vi "HP 3458A Utility Output Format.vi"(5 "Output Format (0:ASCII)":T1(ring), 7 "Numbers of Reading (1)":i32=1, 9 "Input String":string) -> (4 "Output Data (ASCII)":dbl[](array[numeric]) format="%.4e", 6 "Output Data (Double Real)":dbl[](array[numeric]) format="%.4e", 8 "Output Data (Single Real)":sgl[](array[numeric]) format="%.4e", 10 "Output Data (Single Integer)":i16[](array[numeric]), 15 "Output Data (Double Integer)":i32[](array[numeric]) format="%.4e")   [LabVIEW 2014, in "SamplerPlugins.lvlib" / "HP3458aDMM.lvclass"]
doc: "This VI takes an input string and converts the string into numeric value according to the type of data that are being sent back. If the data type is not in ASCII characters, typecasting is then performed to changes the string into numeric type, with each number stored as an element in the output array."
uses:
  HP3458aDMM.lvclass
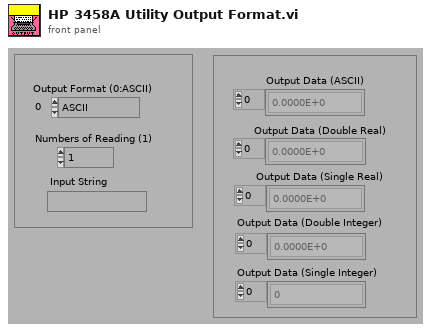
[diagram p1: front panel]
types:
  T1 = enum16{"ASCII", "Single Real", "Double Real", "Single Integer", "Double Integer"}
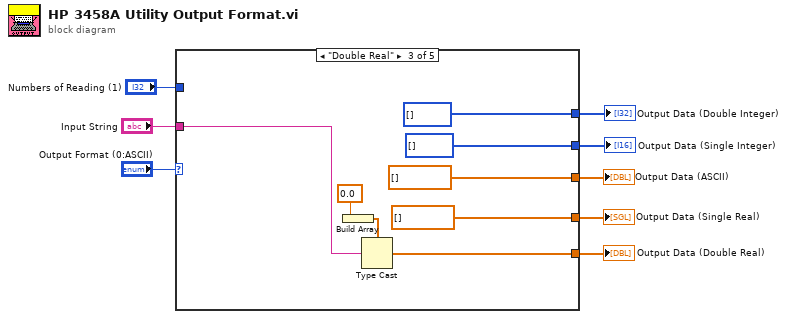
[diagram p0: block diagram]
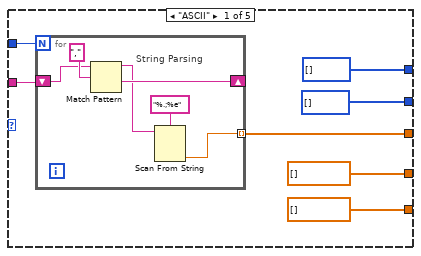
[diagram p2: hidden frame]
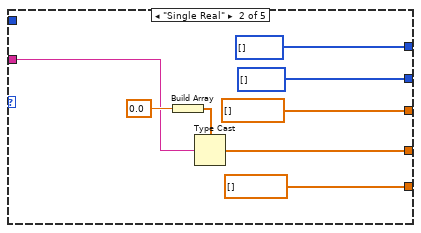
[diagram p3: hidden frame]
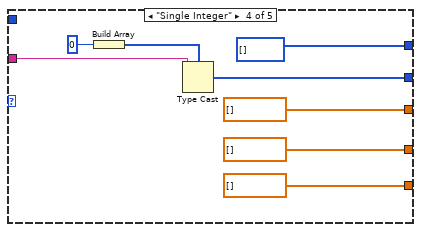
[diagram p4: hidden frame]
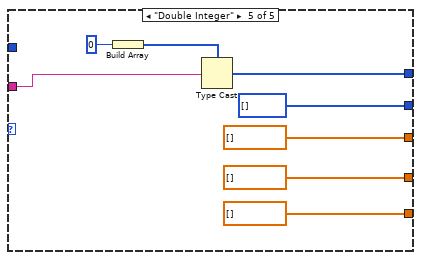
[diagram p5: hidden frame]
diagram:
  n1 = case shown="\"Double Real\"" "Output Format (0:ASCII)" {
    tunnel: [dbl[] [] dbl[] [] w35 dbl[] [] dbl[] []] -> w4
    tunnel: [sgl[] [] w26 sgl[] [] sgl[] [] sgl[] []] -> w5
    tunnel: [w15 dbl[] [] dbl[] [] dbl[] [] dbl[] []] -> w6
    tunnel: "Input String" -> [w9 w24 w32 w44 w51]
    tunnel: "Numbers of Reading (1)" -> [w14 _ _ _ _]
    tunnel: [i8[] [] i8[] [] i8[] [] w39 i8[] []] -> w2
    tunnel: [i16[] [] i16[] [] i16[] [] i16[] [] w46] -> w1
    frame "ASCII" {
      n2 = for {
        N: w14 -> [_]
        tunnel: [w20] -> w15 mode=indexing
        shift-right: [w18] -> _
        shift-left: w9 -> [w17]
        # "String Parsing"
        n3 = Match Pattern(string=w17, regular expression=",") -> (before substring=w16:string, after substring=w18:string)  [unwired: 1 in, 2 out]
        n4 = Scan From String(format string="%.;%e", input string=w16) -> (output 1=w20:dbl)  [unwired: 3 in, 3 out]
      }
    }
    frame "Single Real" {
      n5 = Build Array(sgl 0.0 ("single floating point representation")) -> (w29:sgl[])
      n6 = Type Cast(type=w29, x=w24) -> (*(type *) &x=w26:sgl[])
    }
    frame "Double Real" {
      n7 = Build Array(0.0 ("double floating point representation")) -> (w37:dbl[])
      n8 = Type Cast(type=w37, x=w32) -> (*(type *) &x=w35:dbl[])
    }
    frame "Single Integer" {
      n9 = Build Array(i16 0 ("word integer representation")) -> (w45:i16[])
      n10 = Type Cast(type=w45, x=w44) -> (*(type *) &x=w39:i16[])
    }
    frame "Double Integer" {
      n11 = Build Array(0 ("long integer representation")) -> (w53:i32[])
      n12 = Type Cast(type=w53, x=w51) -> (*(type *) &x=w46:i32[])
    }
  }
  "Output Data (ASCII)" <- w6
  "Output Data (Single Real)" <- w5
  "Output Data (Double Real)" <- w4
  "Output Data (Single Integer)" <- w2
  "Output Data (Double Integer)" <- w1
